vi "Read font size (15).vi"(8 "error in (no error)":errorcluster, 11 "control label adjustment in":refnum<class "control label adjustment.lvclass">) -> (0 "error out":errorcluster, 2 "font size (15)":u32=15, 3 "control label adjustment out":refnum<class "control label adjustment.lvclass">)   [LabVIEW 2013, in "control label adjustment.lvclass"]
uses:
  control label adjustment.lvclass
  control label adjustment.lvclass/control label adjustment.ctl
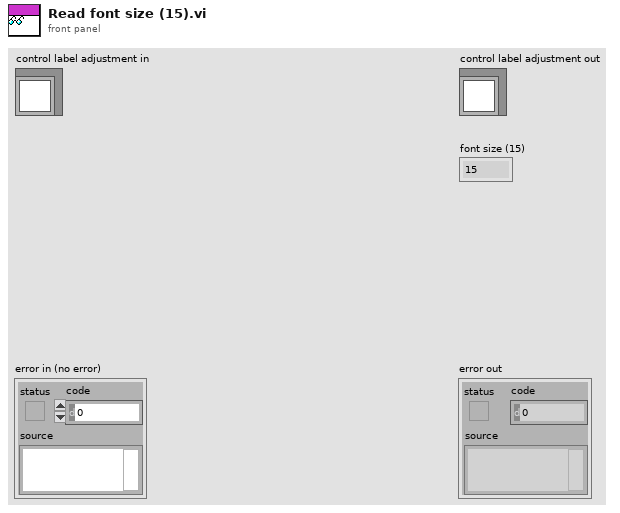
[diagram p1: front panel]
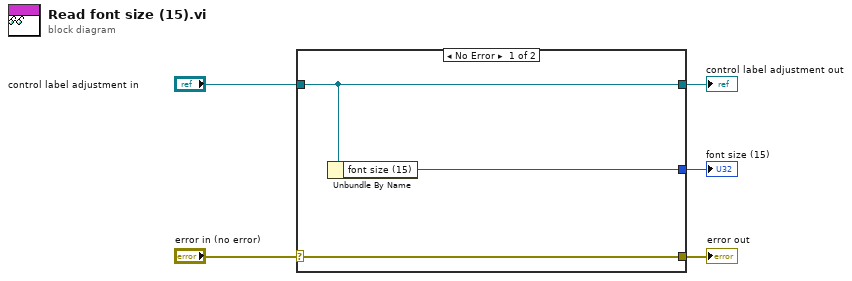
[diagram p0: block diagram]
diagram:
  n1 = case shown="No Error" "error in (no error)" {
    selector: "error in (no error)" -> [w8 w9]
    tunnel: [w8 w9] -> w4
    tunnel: [w7 w10] -> w2
    tunnel: "control label adjustment in" -> [w7 w10]
    tunnel: [w6 _] -> w1
    frame No Error {
      n2 = Unbundle By Name(w7) -> ("font size (15)"=w6:u32)
    }
    frame Error {
    }
  }
  "error out" <- w4
  "control label adjustment out" <- w2
  "font size (15)" <- w1
